vi "Waveform-Processing-Custom-Device.Async.vi"(10 "Parameters":variant, 11 "Process":refnum<class "Process.lvclass">) -> ()   [LabVIEW 2020, in "Waveform-Processing-Custom-Device Engine.lvlib"]
uses:
  Waveform-Processing-Custom-Device Engine.lvlib
  <vilib>/NI/NIVS Inline Async API/_VS Inline Async API/Process/Process.lvclass
  Shared/Running Average/Running Average.lvlib
  Shared/Single Point/SinglePoint.lvlib
  <vilib>/NI VeriStand/Custom Device API/Data Reference.ctl
  <vilib>/NI VeriStand/Custom Device API/Custom Device API.lvlib
  <vilib>/NI VeriStand/Custom Device API/Block Data Reference.ctl
  <vilib>/NI VeriStand/Custom Device API/Waveform Data Reference.ctl
  Shared/CompiledSettings.ctl
  Shared/Waveform-Processing-Custom-Device Shared.lvlib
  Shared/Scaled Waveform/Scaled Waveform.lvlib
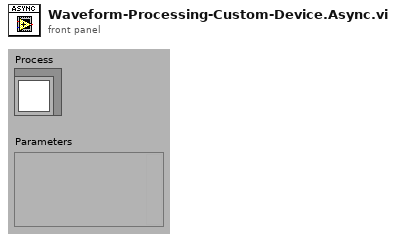
[diagram p1: front panel]
types:
  T1 = typedef "Waveform-Processing-Custom-Device Shared.lvlib/CompiledSettings.ctl" = cluster{"Name":string, "Buffer Length (samples)":u32, "Enable Array":bool[], "Parameter Block Data Refs":T2[], "Source Wfm Data Refs":T4[], "Result Wfm Data Refs":T4[], "Result Ch Data Refs":T3[], "Task Rate (Hz)":dbl}
  T2 = typedef "Custom Device API.lvlib/Block Data Reference.ctl" = cluster{"Data Reference":T3, "Offset":u64, "Length":u64}
  T3 = typedef "Custom Device API.lvlib/Data Reference.ctl" = i32
  T4 = typedef "Custom Device API.lvlib/Waveform Data Reference.ctl" = i32
  T5 = typedef "Waveform-Processing-Custom-Device Engine.lvlib/AsyncStateVariables.ctl" = cluster{"Source Wfm Session Refs":refnum<class "Single Waveform Read (DBL).lvclass">[], "Result Wfm Session Refs":refnum<class "Single Waveform Write (DBL).lvclass">[], "Result Wfm Data":dbl[][], "Source Wfm Data Refs":T4[], "Result Wfm Data Refs":T4[], "Global Buffer Length (samples)":dbl, "Parameter Array":dbl[], "Tag Results":dbl[], "Enable Array":bool[], "Task Rate":dbl, "Data FIFO Refs":cluster{"Single Point Result":T6, "Running Average Result":T6, "Running Average Parameters":T7, "Scaled Waveform Parameters":T7}}
  T6 = typedef "Data Access Engine.lvlib/Data Access Engine.lvclass/Write.DVR.ctl" = refnum<data-value>
  T7 = typedef "Data Access Engine.lvlib/Data Access Engine.lvclass/Read.DVR.ctl" = refnum<data-value>
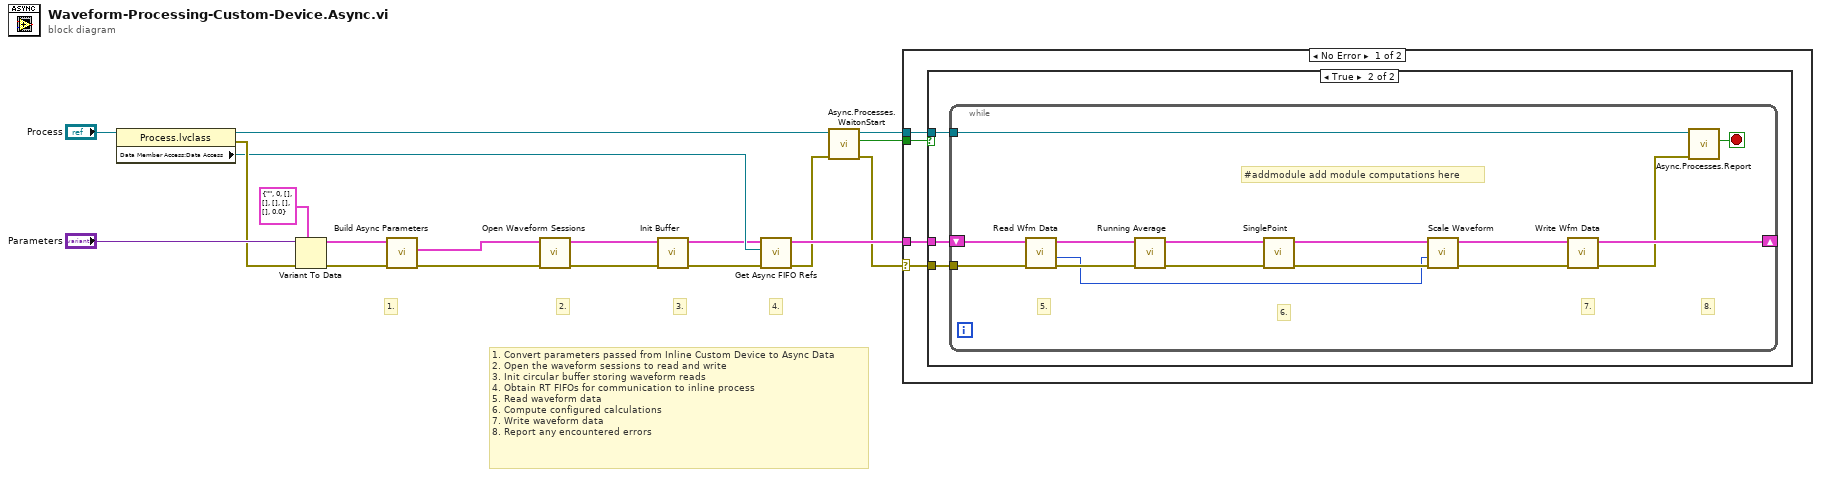
[diagram p0: block diagram]
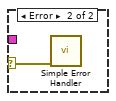
[diagram p3: hidden frame]
diagram:
  # "4."
  # "3."
  # "2."
  # "1."
  # "1. Convert parameters passed from Inline Custom Device to Async Data\n2. Open the waveform sessions to read and write\n3. Init circular buffer storing waveform reads\n4. Obtain RT FIFOs for communication to inline process\n5. Read waveform data\n6. Compute configured calculations\n7. Write waveform data\n8. Report any encountered errors"
  n1 = property class="Process.lvclass"(reference="Process") -> (reference out=w16:refnum<class "Process.lvclass">, error out=w14:errorcluster, "Data Member Access:Data Access"=w12:refnum<class "Data Access Engine.lvclass">)  [unwired: 1 in]
  n2 = Variant To Data(error in=w14, type=T1 {"Name"="", "Buffer Length (samples)"=0, "Enable Array"=[], "Parameter Block Data Refs"=[], "Source Wfm Data Refs"=[], "Result Wfm Data Refs"=[], "Result Ch Data Refs"=[], "Task Rate (Hz)"=0.0} ("CompiledSettings"), Variant="Parameters") -> (data=w6:T1, error out=w8:errorcluster)
  n3 = call "Build Async Parameters.vi"("Error in"=w8, "CompiledSettings In"=w6) -> ("Error out"=w1:errorcluster, "Async State Vars"=w7:T5)  [unwired: 7 in, 1 out]
  n4 = call "Open Waveform Sessions.vi"("error in"=w1, "Async State Vars"=w7) -> ("error out"=w3:errorcluster, "Async State Vars out"=w13:T5)  [unwired: 8 in]
  n5 = call "Init Buffer.vi"("Error in"=w3, "Async State Vars"=w13) -> ("Error out"=w2:errorcluster, "Async State Vars out"=w11:T5)  [unwired: 8 in]
  n6 = call "Get Async FIFO Refs.vi"("error in (no error)"=w2, "Data Access API In"=w12, "Async State Vars In"=w11) -> ("error out"=w5:errorcluster, "Async State Vars Out"=w10:T5)  [unwired: 6 in, 1 out]
  n7 = call <vilib>:"Async.Processes.WaitonStart.vi"("error in (no error)"=w5, "Process"=w16) -> ("error out"=w4:errorcluster, "Execute"=w19:bool, "Process out"=w18:refnum<class "Process.lvclass">)  [unwired: 7 in]
  n8 = case shown="No Error" w4 {
    selector: w4 -> [w21 w42]
    tunnel: w19 -> [w23 _]
    tunnel: w18 -> [w22 _]
    tunnel: w10 -> [w20 _]
    frame No Error {
      n9 = case shown="True" w23 {
        tunnel: w21 -> [_ w25]
        tunnel: w22 -> [_ w26]
        tunnel: w20 -> [_ w24]
        frame False {
        }
        frame True {
          n10 = while {
            tunnel: w25 -> [w32]
            tunnel: w26 -> [w41]
            shift-right: [w37] -> _
            shift-left: w24 -> [w39]
            stop <- w40 stop-if-true
            # "#addmodule add module computations here"
            # "8."
            # "7."
            # "6."
            # "5."
            n11 = call "Read Wfm Data.vi"("error in (no error)"=w32, "Async State Vars in"=w39) -> ("error out"=w35:errorcluster, "samples read"=w27:i32, "Async State Vars out"=w38:T5)  [unwired: 6 in, 1 out]
            n12 = call "Running Average.vi"("Error In"=w35, "Async State Vars 2"=w38) -> ("Error Out"=w34:errorcluster, "Async State Vars out"=w36:T5)  [unwired: 8 in]
            n13 = call "SinglePoint.vi"("Error In 2"=w34, "Async State Vars 2"=w36) -> ("Error Out"=w31:errorcluster, "Async State Vars out"=w30:T5)  [unwired: 8 in]
            n14 = call "Scale Waveform.vi"("Error In"=w31, "Read Size"=w27, "Async State Vars 2"=w30) -> ("Error Out"=w29:errorcluster, "Async State Vars out"=w28:T5)  [unwired: 7 in]
            n15 = call "Write Wfm Data.vi"("error in (no error)"=w29, "Async State Vars in"=w28) -> ("error out"=w33:errorcluster, "Async State Vars out"=w37:T5)  [unwired: 7 in, 1 out]
            n16 = call <vilib>:"Async.Processes.Report.vi"("Error"=w33, "Process in"=w41) -> ("Stop"=w40:bool)  [unwired: 8 in, 1 out]
          }
        }
      }
    }
    frame Error {
      n17 = call <vilib>:"Simple Error Handler.vi"("error in (no error)"=w42) -> ()  [unwired: 4 in, 5 out]
    }
  }
